vi "CalcTSR.vi"(9 "WindSpeed":dbl, 10 "SimulationConst":T1={"Ngear"=0.0, "RotorInertia"=0.0, "GeneratorEff"=0.0, "RotorRadius"=0.0, "Rho"=0.9700000286102295, "NumBlades"=1, "ScaleFactor"=3.0}, 11 "GenSpeed":dbl) -> (2 "SimulationConst Out":T1={"Ngear"=0.0, "RotorInertia"=0.0, "GeneratorEff"=0.0, "RotorRadius"=0.0, "Rho"=0.9700000286102295, "NumBlades"=1, "ScaleFactor"=3.0}, 3 "TSR":dbl)   [LabVIEW 2018]
uses:
  Clusters/SimulationConstants.ctl
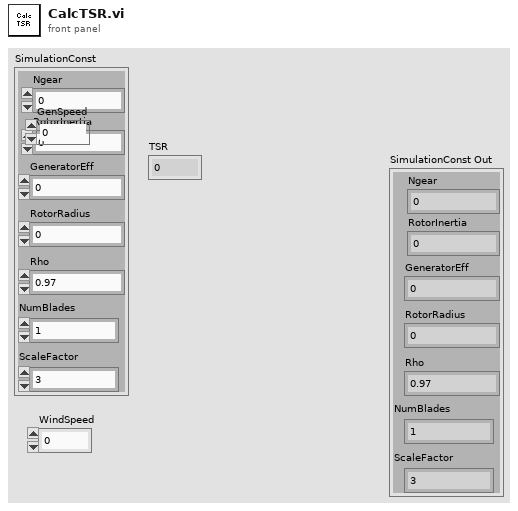
[diagram p1: front panel]
types:
  T1 = typedef "SimulationConstants.ctl" = cluster{"Ngear":dbl, "RotorInertia":dbl, "GeneratorEff":dbl, "RotorRadius":sgl, "Rho":dbl, "NumBlades":i32, "ScaleFactor":dbl}
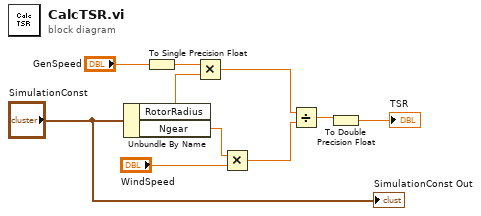
[diagram p0: block diagram]
diagram:
  n1 = Unbundle By Name("SimulationConst") -> ("RotorRadius"=w5:sgl, "Ngear"=w6:dbl)
  n2 = To Single Precision Float(number="GenSpeed") -> (single precision float=w3:sgl)
  n3 = Multiply(x=w3, y=w5) -> (x*y=w7:sgl)
  n4 = Multiply(x=w6, y="WindSpeed") -> (x*y=w8:dbl)
  n5 = Divide(x=w7, y=w8) -> (x/y=w10:dbl)
  n6 = To Double Precision Float(number=w10) -> (double precision float=→"TSR":dbl)
  "SimulationConst Out" <- "SimulationConst"
